vi "loadcontrsval.vi"(4 "error in":errorcluster, 5 "Array":refnum<vi>[](array[refnum]), 6 "Section":string, 7 "refnum in":T1) -> (0 "error out":errorcluster, 1 "Array 2":string[][](array[string]), 3 "refnum out":T1)   [LabVIEW 2010]
uses:
  <vilib>/Utility/config.llb/Config Data RefNum.ctl
  <vilib>/Utility/config.llb/Read Key (String).vi
  <vilib>/Utility/config.llb/Write Key (String).vi
  <vilib>/Utility/config.llb/Read Key (Path).vi
  <vilib>/Utility/config.llb/Write Key (Path).vi
  <vilib>/Utility/config.llb/Read Key (Double).vi
  <vilib>/Utility/config.llb/Write Key (Double).vi
  <vilib>/Utility/config.llb/Read Key (Boolean).vi
  <vilib>/Utility/config.llb/Write Key (Boolean).vi
  <vilib>/Utility/config.llb/NI_LVConfig.lvlib
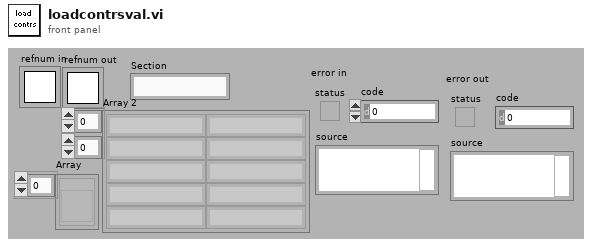
[diagram p1: front panel]
types:
  T1 = typedef "NI_LVConfig.lvlib/Config Data RefNum.ctl" = refnum<k1>
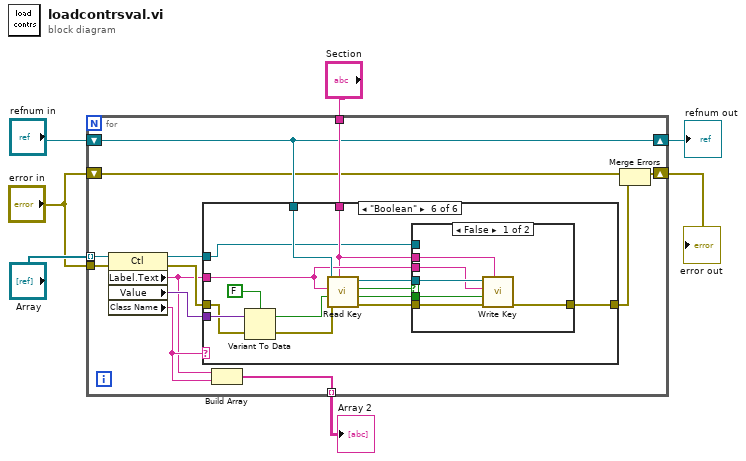
[diagram p0: block diagram]
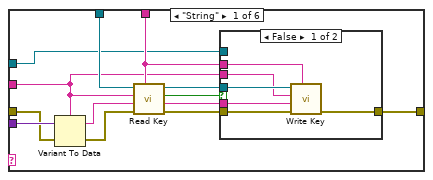
[diagram p2: hidden frame]
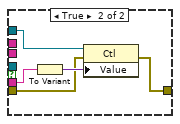
[diagram p3: hidden frame]
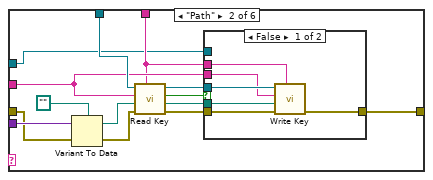
[diagram p4: hidden frame]
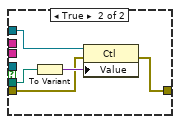
[diagram p5: hidden frame]
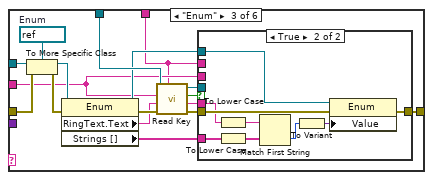
[diagram p6: hidden frame]
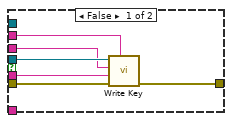
[diagram p7: hidden frame]
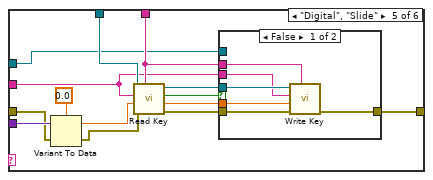
[diagram p9: hidden frame]
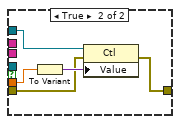
[diagram p10: hidden frame]
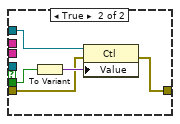
[diagram p11: hidden frame]
diagram:
  n1 = for {
    tunnel: "Section" -> [w18]
    tunnel: "Array" -> [w20] mode=indexing
    shift-right: [w16] -> w7
    shift-left: "refnum in" -> [w16]
    shift-right: [w12] -> w3
    shift-left: "error in" -> [w13]
    tunnel: "error in" -> [w14]
    tunnel: [w9] -> w1 mode=indexing
    n2 = property on="Property Node" class="Ctl"(reference=w20, error in=w14) -> (reference out=w17:refnum<vi>, error out=w15:errorcluster, "Label.Text"=w10:string, "Value"=w19:variant, "Class Name"=w11:string)
    n3 = case shown="\"Boolean\"" w11 {
      tunnel: w19 -> [w33 w58 _ _ w116 w141]
      tunnel: w18 -> [w23 w46 w72 _ w105 w129]
      tunnel: w16 -> [w31 w56 w84 _ w113 w139]
      tunnel: w10 -> [w22 w47 w73 _ w104 w130]
      tunnel: w17 -> [w21 w45 w83 _ w103 w128]
      tunnel: w15 -> [w30 w54 w81 w102 w112 w137]
      tunnel: [w27 w52 w79 w102 w110 w135] -> w8
      frame "String" {
        n4 = Variant To Data(error in=w30, Variant=w33, type=w22) -> (error out=w29:errorcluster, data=w32:string)
        n5 = call-poly <vilib>:"Read Key.vi"("section"=w23, "error in (no error)"=w29, "default value"=w32, "key"=w22, "refnum"=w31) -> ("error out"=w28:errorcluster, "value"=w24:string, "found?"=w26:bool, "refnum out"=w25:T1)  [unwired: 3 in]
        n6 = case shown="False" w26 {
          tunnel: w23 -> [w39 _]
          tunnel: w28 -> [w38 w41]
          tunnel: [w37 w40] -> w27
          tunnel: w25 -> [w36 _]
          tunnel: w22 -> [w35 _]
          tunnel: w24 -> [w34 w44]
          tunnel: w21 -> [_ w42]
          frame False {
            n7 = call-poly <vilib>:"Write Key.vi"("section"=w39, "error in (no error)"=w38, "value"=w34, "key"=w35, "refnum"=w36) -> ("error out"=w37:errorcluster)  [unwired: 4 in, 2 out]
          }
          frame True {
            n8 = To Variant(anything=w44) -> (Variant=w43:variant)
            n9 = property class="Ctl"(reference=w42, error in=w41, "Value"=w43) -> (error out=w40:errorcluster)  [unwired: 1 out]
          }
        }
      }
      frame "Path" {
        n10 = Variant To Data(error in=w54, Variant=w58, type=path "") -> (error out=w53:errorcluster, data=w57:path)
        n11 = call-poly <vilib>:"Read Key.vi"("section"=w46, "error in (no error)"=w53, "default value"=w57, "key"=w47, "refnum"=w56) -> ("error out"=w51:errorcluster, "value"=w50:path, "found?"=w49:bool, "refnum out"=w48:T1)  [unwired: 3 in]
        n12 = case shown="False" w49 {
          tunnel: w46 -> [w64 _]
          tunnel: w51 -> [w63 w66]
          tunnel: [w62 w65] -> w52
          tunnel: w48 -> [w61 _]
          tunnel: w47 -> [w60 _]
          tunnel: w50 -> [w59 w69]
          tunnel: w45 -> [_ w67]
          frame False {
            n13 = call-poly <vilib>:"Write Key.vi"("section"=w64, "error in (no error)"=w63, "value"=w59, "key"=w60, "refnum"=w61) -> ("error out"=w62:errorcluster)  [unwired: 4 in, 2 out]
          }
          frame True {
            n14 = To Variant(anything=w69) -> (Variant=w68:variant)
            n15 = property class="Ctl"(reference=w67, error in=w66, "Value"=w68) -> (error out=w65:errorcluster)  [unwired: 1 out]
          }
        }
      }
      frame "Enum" {
        w86 = refnum<vi> refnum  # Enum
        n16 = To More Specific Class(target class=w86, reference=w83, error in=w81) -> (specific class reference=w85:refnum<vi>, error out=w80:errorcluster)
        n17 = property class="Enum"(reference=w85, error in=w80) -> (reference out=w76:refnum<vi>, error out=w82:errorcluster, "RingText.Text"=w70:string, "Strings []"=w71:string[])
        n18 = call-poly <vilib>:"Read Key.vi"("section"=w72, "error in (no error)"=w82, "default value"=w70, "key"=w73, "refnum"=w84) -> ("error out"=w78:errorcluster, "value"=w77:string, "found?"=w75:bool, "refnum out"=w74:T1)  [unwired: 3 in]
        n19 = case shown="True" w75 {
          tunnel: w72 -> [w92 _]
          tunnel: w78 -> [w91 w99]
          tunnel: [w90 w98] -> w79
          tunnel: w74 -> [w89 _]
          tunnel: w73 -> [w88 _]
          tunnel: w77 -> [w87 w96]
          tunnel: w76 -> [_ w100]
          tunnel: w71 -> [_ w97]
          frame False {
            n20 = call-poly <vilib>:"Write Key.vi"("section"=w92, "error in (no error)"=w91, "value"=w87, "key"=w88, "refnum"=w89) -> ("error out"=w90:errorcluster)  [unwired: 4 in, 2 out]
          }
          frame True {
            n21 = To Lower Case(string=w96) -> (all lower case string=w93:string)
            n22 = To Lower Case(string=w97) -> (all lower case string=w94:string[])
            n23 = Match First String(2:w94, 3:w93) -> (0:w95:i32)  [unwired: 1 out]
            n24 = To Variant(anything=w95) -> (Variant=w101:variant)
            n25 = property class="Enum"(reference=w100, error in=w99, "Value"=w101) -> (error out=w98:errorcluster)  [unwired: 1 out]
          }
        }
      }
      frame "Any", Default {
      }
      frame "Digital", "Slide" {
        n26 = Variant To Data(error in=w112, Variant=w116, type=0.0 ("number")) -> (error out=w111:errorcluster, data=w114:dbl)
        n27 = call-poly <vilib>:"Read Key.vi"("section"=w105, "error in (no error)"=w111, "default value"=w114, "key"=w104, "refnum"=w113) -> ("error out"=w109:errorcluster, "value"=w108:dbl, "found?"=w107:bool, "refnum out"=w106:T1)  [unwired: 3 in]
        n28 = case shown="False" w107 {
          tunnel: w105 -> [w122 _]
          tunnel: w109 -> [w121 w124]
          tunnel: [w120 w123] -> w110
          tunnel: w106 -> [w119 _]
          tunnel: w104 -> [w118 _]
          tunnel: w108 -> [w117 w127]
          tunnel: w103 -> [_ w125]
          frame False {
            n29 = call-poly <vilib>:"Write Key.vi"("section"=w122, "error in (no error)"=w121, "value"=w117, "key"=w118, "refnum"=w119) -> ("error out"=w120:errorcluster)  [unwired: 4 in, 2 out]
          }
          frame True {
            n30 = To Variant(anything=w127) -> (Variant=w126:variant)
            n31 = property class="Ctl"(reference=w125, error in=w124, "Value"=w126) -> (error out=w123:errorcluster)  [unwired: 1 out]
          }
        }
      }
      frame "Boolean" {
        n32 = Variant To Data(error in=w137, Variant=w141, type=FALSE) -> (error out=w136:errorcluster, data=w140:bool)
        n33 = call-poly <vilib>:"Read Key.vi"("section"=w129, "error in (no error)"=w136, "default value"=w140, "key"=w130, "refnum"=w139) -> ("error out"=w134:errorcluster, "value"=w133:bool, "found?"=w132:bool, "refnum out"=w131:T1)  [unwired: 3 in]
        n34 = case shown="False" w132 {
          tunnel: w129 -> [w147 _]
          tunnel: w134 -> [w146 w149]
          tunnel: [w145 w148] -> w135
          tunnel: w131 -> [w144 _]
          tunnel: w130 -> [w143 _]
          tunnel: w133 -> [w142 w152]
          tunnel: w128 -> [_ w150]
          frame False {
            n35 = call-poly <vilib>:"Write Key.vi"("section"=w147, "error in (no error)"=w146, "value"=w142, "key"=w143, "refnum"=w144) -> ("error out"=w145:errorcluster)  [unwired: 4 in, 2 out]
          }
          frame True {
            n36 = To Variant(anything=w152) -> (Variant=w151:variant)
            n37 = property class="Ctl"(reference=w150, error in=w149, "Value"=w151) -> (error out=w148:errorcluster)  [unwired: 1 out]
          }
        }
      }
    }
    n38 = Build Array(w10, w11) -> (w9:string[])
    n39 = Merge Errors(w13, w8) -> (w12:errorcluster)
  }
  "refnum out" <- w7
  "error out" <- w3
  "Array 2" <- w1
